vi "Initialize Monitor.vi"(8 "error in (no error)":errorcluster, 10 "Target Ref in":T8 format="%.0x", 11 "Addon Ref in":T8 format="%.0x") -> (0 "error out":errorcluster, 2 "Found?":bool, 3 "Monitor Frame Configurations":T1[](array[typedef]) {"Validation Channels Refs"."Data Reference" format="%.0x"; "CD Results Refs"."Data Reference" format="%.0x"; "Input Channels Refs"."Data Reference" format="%.0x"; "Frame Configuration"."CRCConfiguration"."FinalXorValue" format="%0x"; "Frame Configuration"."CRCConfiguration"."InitialCRC" format="%0x"; "Frame Configuration"."CRCConfiguration"."Polynomial" format="%0x"; "Frame Configuration"."CRC"."Data Type" items=["Signed", "Unsigned", "IEEE Float"]; "Frame Configuration"."Rolling Counter"."Data Type" items=["Signed", "Unsigned", "IEEE Float"]; "Frame Configuration"."Input Channels"."Data Type" items=["Signed", "Unsigned", "IEEE Float"]})   [LabVIEW 2021, in "LIN Frame Protection Addon Engine.lvlib"]
uses:
  LIN Frame Protection Addon Engine.lvlib
  <vilib>/NI VeriStand/Custom Device API/Custom Device Item Ref.ctl
  Types/RT Engine Monitor References.ctl
  Shared/Types/FrameConfiguration.ctl
  Shared/Types/InputChannelConfiguration.ctl
  Shared/Types/Protection Type.ctl
  Shared/Types/CRCConfiguration.ctl
  <vilib>/NI VeriStand/Custom Device API/Block Data Reference.ctl
  <vilib>/NI VeriStand/Custom Device API/Data Reference.ctl
  <vilib>/NI VeriStand/Custom Device Tools/Custom Device Utility Library/Search Direction.ctl
  <vilib>/NI VeriStand/Custom Device API/Data Access Type.ctl
  Shared/SubVIs/GUID Lookup.vi
  <vilib>/NI VeriStand/Custom Device Tools/Custom Device Utility Library/NI VeriStand - Search for Item by GUID.vi
  <vilib>/NI VeriStand/Custom Device Tools/Custom Device Utility Library/NI VeriStand - Search for All Items by GUID.vi
  <vilib>/xnet/xnet.llb/XNET Create Session (Conversion).vi
  <vilib>/NI VeriStand/Custom Device Tools/Custom Device Utility Library/Custom Device Utility Library.lvlib
  Shared/LIN Frame Protection Addon Shared.lvlib
  <vilib>/NI VeriStand/Custom Device API/Custom Device API.lvlib
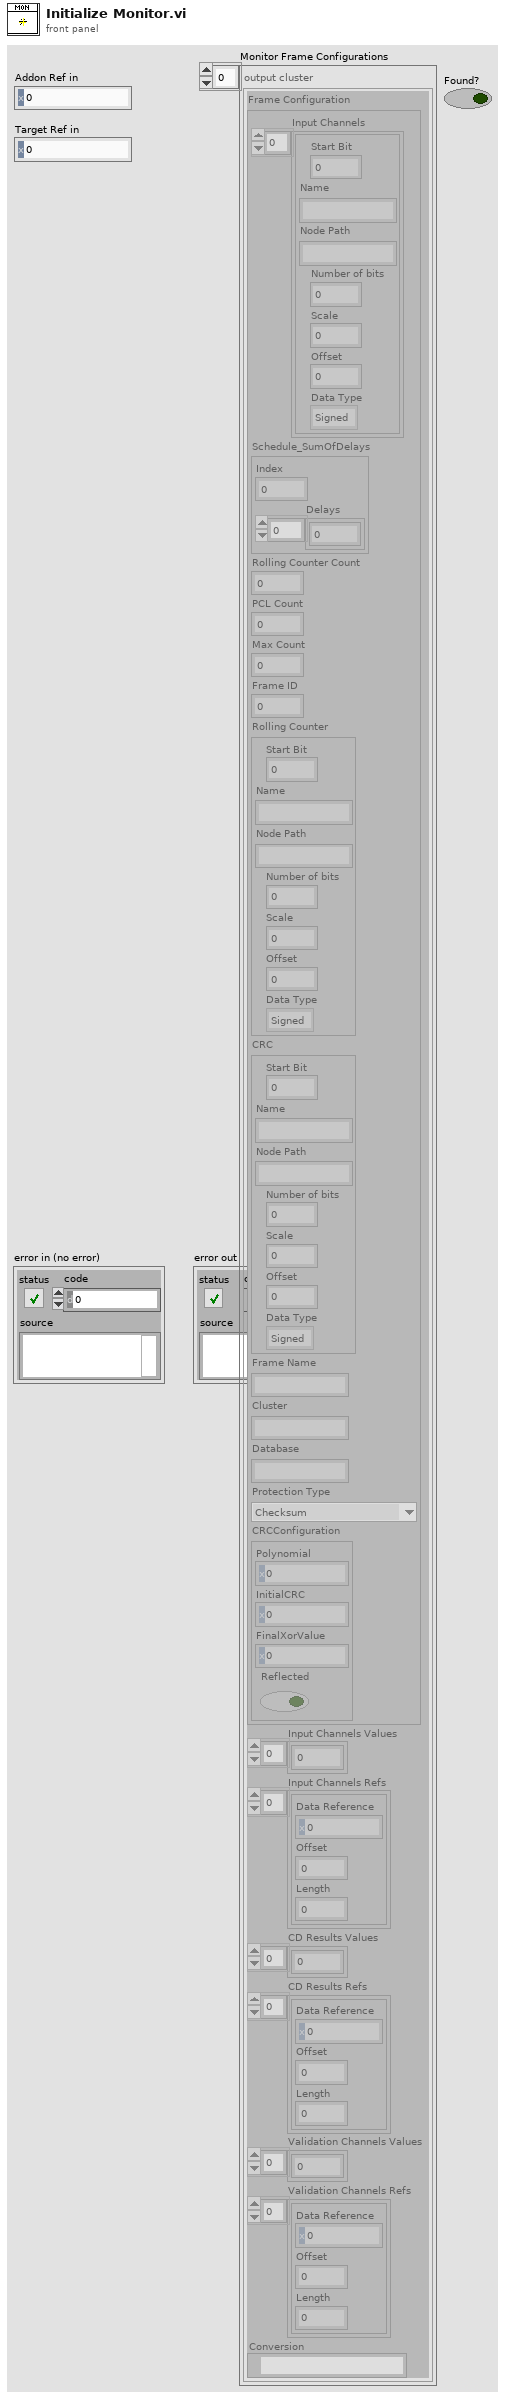
[diagram p1: front panel]
types:
  T1 = typedef "LIN Frame Protection Addon Engine.lvlib/RT Engine Monitor References.ctl" = cluster{"Frame Configuration":T2, "Input Channels Values":dbl[], "Input Channels Refs":T6[], "CD Results Values":dbl[], "CD Results Refs":T6[], "Validation Channels Values":dbl[], "Validation Channels Refs":T6[], "Conversion":refnum<k21>}
  T2 = typedef "LIN Frame Protection Addon Shared.lvlib/FrameConfiguration.ctl" = cluster{"Input Channels":T3[], "Schedule_SumOfDelays":cluster{"Index":i32, "Delays":dbl[]}, "Rolling Counter Count":dbl, "PCL Count":u64, "Max Count":dbl, "Frame ID":u32, "Rolling Counter":T3, "CRC":T3, "Frame Name":string, "Cluster":string, "Database":string, "Protection Type":T4, "CRCConfiguration":T5}
  T3 = typedef "LIN Frame Protection Addon Shared.lvlib/InputChannelConfiguration.ctl" = cluster{"Start Bit":i32, "Name":string, "Node Path":string, "Number of bits":i32, "Scale":dbl, "Offset":dbl, "Data Type":u32}
  T4 = typedef "LIN Frame Protection Addon Shared.lvlib/Protection Type.ctl" = enum16{"Checksum", "CRC-8", "CRC-16", "CRC-32", "None (Counter Only)"}
  T5 = typedef "LIN Frame Protection Addon Shared.lvlib/CRCConfiguration.ctl" = cluster{"Polynomial":u64, "InitialCRC":u64, "FinalXorValue":u64, "Reflected":bool}
  T6 = typedef "Custom Device API.lvlib/Block Data Reference.ctl" = cluster{"Data Reference":T7, "Offset":u64, "Length":u64}
  T7 = typedef "Custom Device API.lvlib/Data Reference.ctl" = i32
  T8 = typedef "Custom Device API.lvlib/Custom Device Item Ref.ctl" = u64
  T9 = typedef "Custom Device Utility Library.lvlib/Search Direction.ctl" = enum16{"Down", "Up"}
  T10 = typedef "Custom Device API.lvlib/Data Access Type.ctl" = enum16{"Read", "Write"}
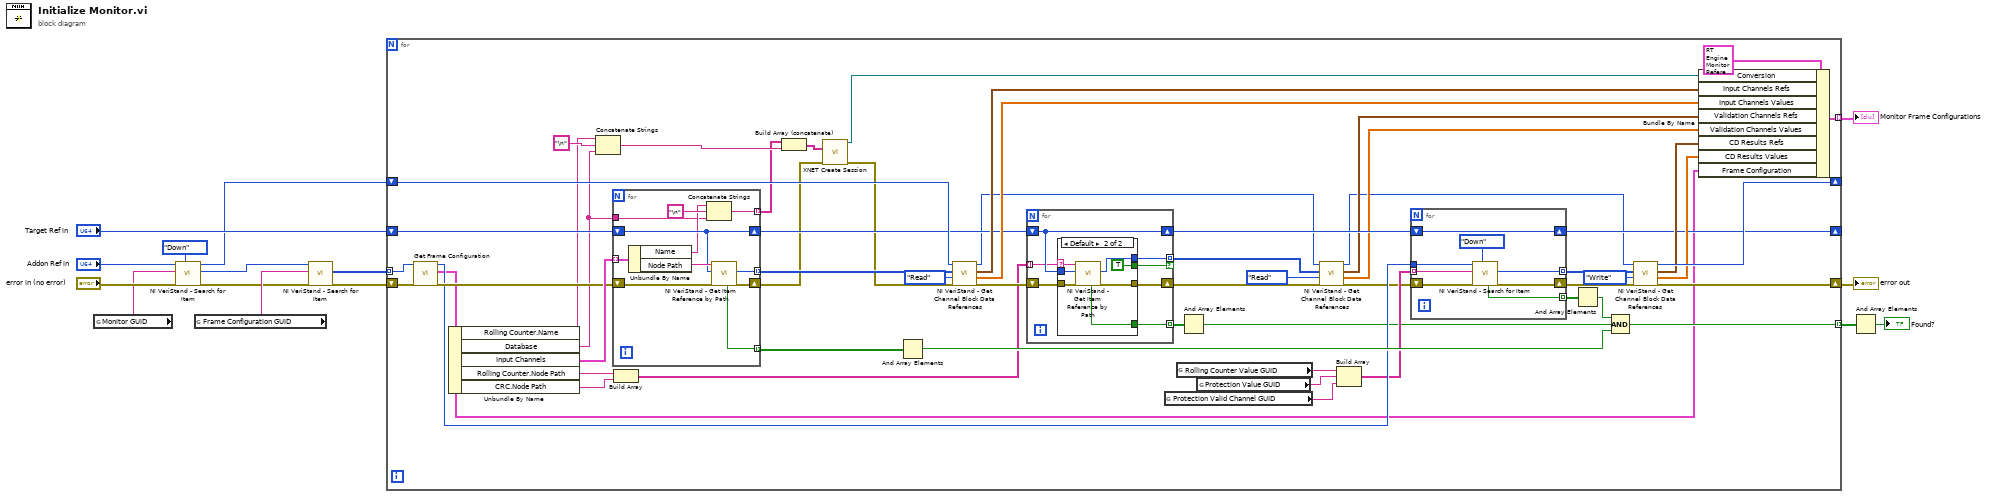
[diagram p0: block diagram]
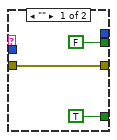
[diagram p2: hidden frame]
diagram:
  n1 = global read "GUID Lookup.vi" "Monitor GUID"() -> (w4:string)
  n2 = call-poly <vilib>:"NI VeriStand - Search for Item.vi"("Direction (Down)"=Search_Direction."Down", "error in"="error in (no error)", "Item GUID"=w4, "Section Ref in"="Addon Ref in") -> ("error out"=w8:errorcluster, "Item Ref"=w6:T8, "Section Ref out"=w5:T8)  [unwired: 4 in, 1 out]
  n3 = global read "GUID Lookup.vi" "Frame Configuration GUID"() -> (w10:string)
  n4 = call-poly <vilib>:"NI VeriStand - Search for Item.vi"("error in"=w8, "Item GUID"=w10, "Section Ref in"=w6) -> ("error out"=w11:errorcluster, "Item Refs"=w12:T8[])  [unwired: 5 in, 2 out]
  n5 = for {
    shift-right: [w52] -> w14
    shift-left: w11 -> [w71]
    tunnel: w12 -> [w70] mode=indexing
    shift-right: [w62] -> _
    shift-left: w5 -> [w49]
    tunnel: [w55] -> w1 mode=indexing
    tunnel: [w57] -> w13 mode=indexing
    shift-right: [w44] -> _
    shift-left: "Target Ref in" -> [w51]
    n6 = call "Get Frame Configuration.vi"("error in"=w71, "Parent Ref"=w70) -> ("error out"=w50:errorcluster, "Selected Channels"=w17:T2, "Parent Ref Out"=w48:T8)  [unwired: 7 in]
    n7 = Unbundle By Name(w17) -> ("Rolling Counter.Name"=w22:string, "Database"=w19:string, "Input Channels"=w69:T3[], "Rolling Counter.Node Path"=w35:string, "CRC.Node Path"=w34:string)
    n8 = Concatenate Strings(w22, "\n" ("string"), w19) -> (w23:string)
    n9 = for {
      tunnel: w69 -> [w107] mode=indexing
      shift-right: [w103] -> w21
      shift-left: w50 -> [w106]
      shift-right: [w101] -> w37
      shift-left: w51 -> [w101]
      tunnel: [w105] -> w65 mode=indexing
      tunnel: [w104] -> w68 mode=indexing
      tunnel: w19 -> [w98]
      tunnel: [w97] -> w18 mode=indexing
      n10 = Unbundle By Name(w107) -> ("Name"=w99:string, "Node Path"=w102:string)
      n11 = Concatenate Strings(w99, "\n" ("string"), w98) -> (w97:string)
      n12 = call <vilib>:"NI VeriStand - Get Item Reference by Path.vi"("error in (no error)"=w106, "Root Ref"=w101, "Item Path in"=w102) -> ("error out"=w103:errorcluster, "Item Ref"=w105:T8, "Found"=w104:bool)  [unwired: 5 in, 1 out]
    }
    n13 = Build Array(w35, w34) -> (w33:string[])
    n14 = Build Array (concatenate)(w18, w23) -> (w25:string[])
    n15 = call-poly <vilib>:"XNET Create Session.vi"("signal list"=w25, "error in (no error)"=w21) -> ("session out"=w16:refnum<k21>, "error out"=w20:errorcluster)  [unwired: 12 out]
    n16 = And Array Elements(Boolean array=w68) -> (logical AND=w67:bool)
    n17 = call <vilib>:"NI VeriStand - Get Channel Block Data References.vi"("error in (no error)"=w20, "Access"=Data_Access_Type."Read", "Channel Refs"=w65, "Device Ref in"=w49) -> ("error out"=w39:errorcluster, "Values Array"=w63:dbl[], "Block Data Refs"=w64:T6[], "Device Ref out"=w28:T8)  [unwired: 4 in]
    n18 = for {
      shift-right: [w75] -> w42
      shift-left: w39 -> [w78]
      shift-right: [w74] -> w36
      shift-left: w37 -> [w74]
      tunnel: [w77] -> w26 mode=indexing if=w72
      tunnel: [w76] -> w40 mode=indexing
      tunnel: w33 -> [w73] mode=indexing
      n19 = case shown="Default" w73 {
        selector: w73 -> [_ w83]
        tunnel: w78 -> [w81 w88]
        tunnel: [_ w87] -> w77
        tunnel: [TRUE ("Found") w86] -> w76
        tunnel: [w81 w85] -> w75
        tunnel: w74 -> [_ w84]
        tunnel: [FALSE TRUE] -> w72
        frame "" {
        }
        frame Default {
          n20 = call <vilib>:"NI VeriStand - Get Item Reference by Path.vi"("error in (no error)"=w88, "Root Ref"=w84, "Item Path in"=w83) -> ("error out"=w85:errorcluster, "Item Ref"=w87:T8, "Found"=w86:bool)  [unwired: 5 in, 1 out]
        }
      }
    }
    n21 = global read "GUID Lookup.vi" "Protection Valid Channel GUID"() -> (w43:string)
    n22 = global read "GUID Lookup.vi" "Rolling Counter Value GUID"() -> (w47:string)
    n23 = And Array Elements(Boolean array=w40) -> (logical AND=w29:bool)
    n24 = global read "GUID Lookup.vi" "Protection Value GUID"() -> (w46:string)
    n25 = call <vilib>:"NI VeriStand - Get Channel Block Data References.vi"("error in (no error)"=w42, "Access"=Data_Access_Type."Read", "Channel Refs"=w26, "Device Ref in"=w28) -> ("error out"=w38:errorcluster, "Values Array"=w30:dbl[], "Block Data Refs"=w31:T6[], "Device Ref out"=w27:T8)  [unwired: 4 in]
    n26 = Build Array(w47, w46, w43) -> (w45:string[])
    n27 = for {
      shift-right: [w94] -> w53
      shift-left: w38 -> [w95]
      shift-right: [w96] -> w44
      shift-left: w36 -> [w96]
      tunnel: [w92] -> w58 mode=indexing
      tunnel: [w93] -> w56 mode=indexing
      tunnel: w48 -> [w91]
      tunnel: w45 -> [w90] mode=indexing
      n28 = call-poly <vilib>:"NI VeriStand - Search for Item.vi"("Direction (Down)"=Search_Direction."Down", "error in"=w95, "Item GUID"=w90, "Section Ref in"=w91) -> ("error out"=w94:errorcluster, "Item Ref"=w92:T8, "Found"=w93:bool)  [unwired: 4 in, 1 out]
    }
    n29 = And Array Elements(Boolean array=w56) -> (logical AND=w54:bool)
    n30 = Compound Arithmetic op=AND(w54, w29, w67) -> (w55:bool)
    n31 = call <vilib>:"NI VeriStand - Get Channel Block Data References.vi"("error in (no error)"=w53, "Access"=Data_Access_Type."Write", "Channel Refs"=w58, "Device Ref in"=w27) -> ("error out"=w52:errorcluster, "Values Array"=w59:dbl[], "Block Data Refs"=w60:T6[], "Device Ref out"=w62:T8)  [unwired: 4 in]
    n32 = Bundle By Name(cluster=T1 {"Frame Configuration"={"Input Channels"=[], "Schedule_SumOfDelays"={"Index"=0, "Delays"=[]}, "Rolling Counter Count"=0.0, "PCL Count"=0, "Max Count"=0.0, "Frame ID"=0, "Rolling Counter"={"Start Bit"=0, "Name"="", "Node Path"="", "Number of bits"=0, "Scale"=0.0, "Offset"=0.0, "Data Type"=0}, "CRC"={"Start Bit"=0, "Name"="", "Node Path"="", "Number of bits"=0, "Scale"=0.0, "Offset"=0.0, "Data Type"=0}, "Frame Name"="", "Cluster"="", "Database"="", "Protection Type"=enum."Checksum", "CRCConfiguration"={"Polynomial"=0, "InitialCRC"=0, "FinalXorValue"=0, "Reflected"=FALSE}}, "Input Channels Values"=[], "Input Channels Refs"=[], "CD Results Values"=[], "CD Results Refs"=[], "Validation Channels Values"=[], "Validation Channels Refs"=[], "Conversion"=""} ("output cluster"), "Conversion"=w16, "Input Channels Refs"=w64, "Input Channels Values"=w63, "Validation Channels Refs"=w31, "Validation Channels Values"=w30, "CD Results Refs"=w60, "CD Results Values"=w59, "Frame Configuration"=w17) -> (w57:T1)
  }
  "error out" <- w14
  "Monitor Frame Configurations" <- w13
  n33 = And Array Elements(Boolean array=w1) -> (logical AND=→"Found?":bool)
